vi "Horst-ECD.vi"() -> ()   [LabVIEW 2017]
uses:
  <vilib>/rvi/interface/nirviMethod/nirviMethod.xnode
  FPGA Bitfiles/HAGAR-VECD_FPGATarget_FPGA-ProgrammECD_J-wKM9Jb3G8.lvbitx
  E:/HAGAR-V_ECD/FPGA-Programm_ECD.vi
  <vilib>/rvi/errors/niLvFpgaMergeErrorWithErrorCode.vi
  <vilib>/FPGAPlugInAG/cRIO-9035/niLvFpga_ReadFifo_cRIO-9035.vi
  <vilib>/FPGAPlugInAG/cRIO-9035/niLvFpga_WriteFifo_cRIO-9035.vi
panel:
  in  "MWAntwortMod2":string[](array[string])=[":0622020121", ":0621020121", ":0626020121", ":0620020121", ":0624020121", ":0625020121", ":0623020121"]
  in  "MWabfragenMod2":string[](array[string])=[":06220401210120", ":06210401210120", ":06260401210120", ":06200401210120", ":06240401210120", ":06250401210120", ":06230401210120"]
  in  "FaktorMod2":dbl[](array[numeric])=[0.00625, 0.00625, 0.15625, 0.00015625, 0.00625, 0.00625, 0.00015625]
  in  "SPvorgebenMod2":string[](array[string])=[":0622010121", ":0621010121", ":0626010121", ":0620010121", ":0624010121", ":0625010121", ":0623010121"]
  in  "FPGA-VI-Referenz":refnum<k20>
  out "Array":errorcluster[](array[cluster])
  out "MW":dbl[](array[numeric])
  out "Fehler":bool[](array[boolean])
  in  "SP":dbl[](array[numeric]) format="%#_13g"
  in  "Stopp":bool
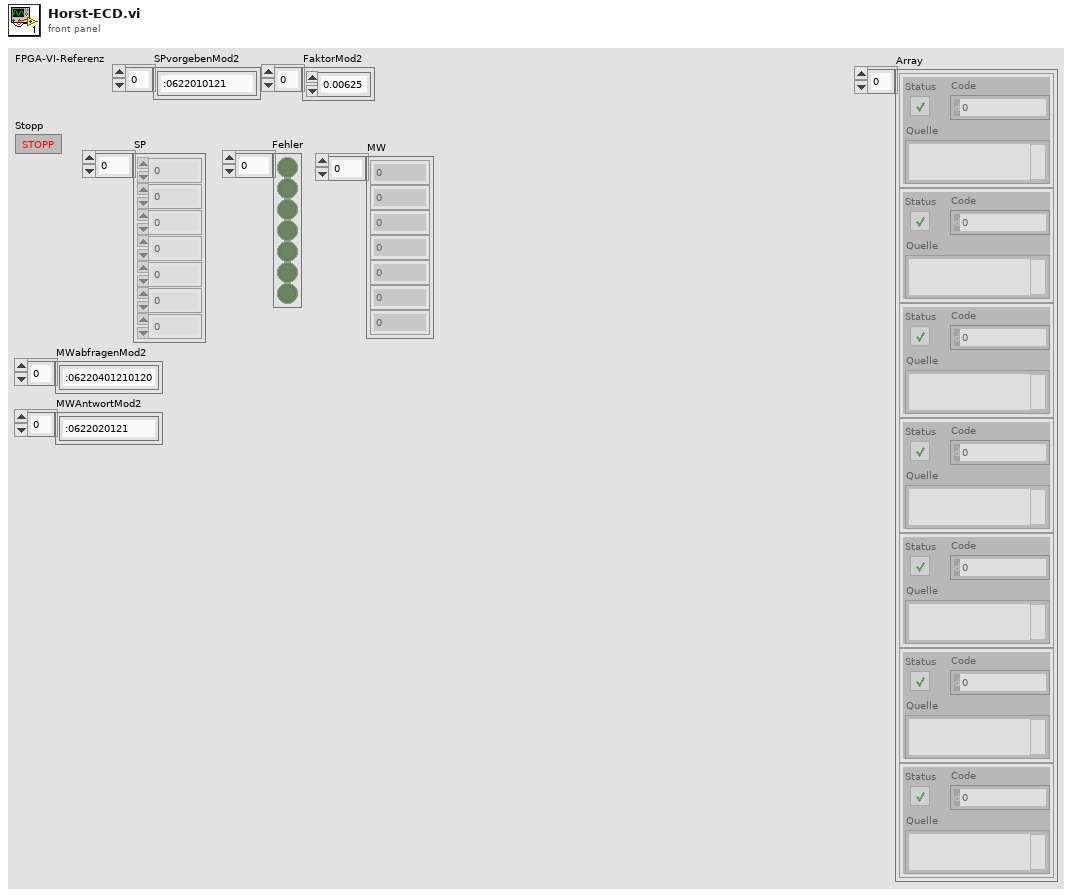
[diagram p1: front panel]
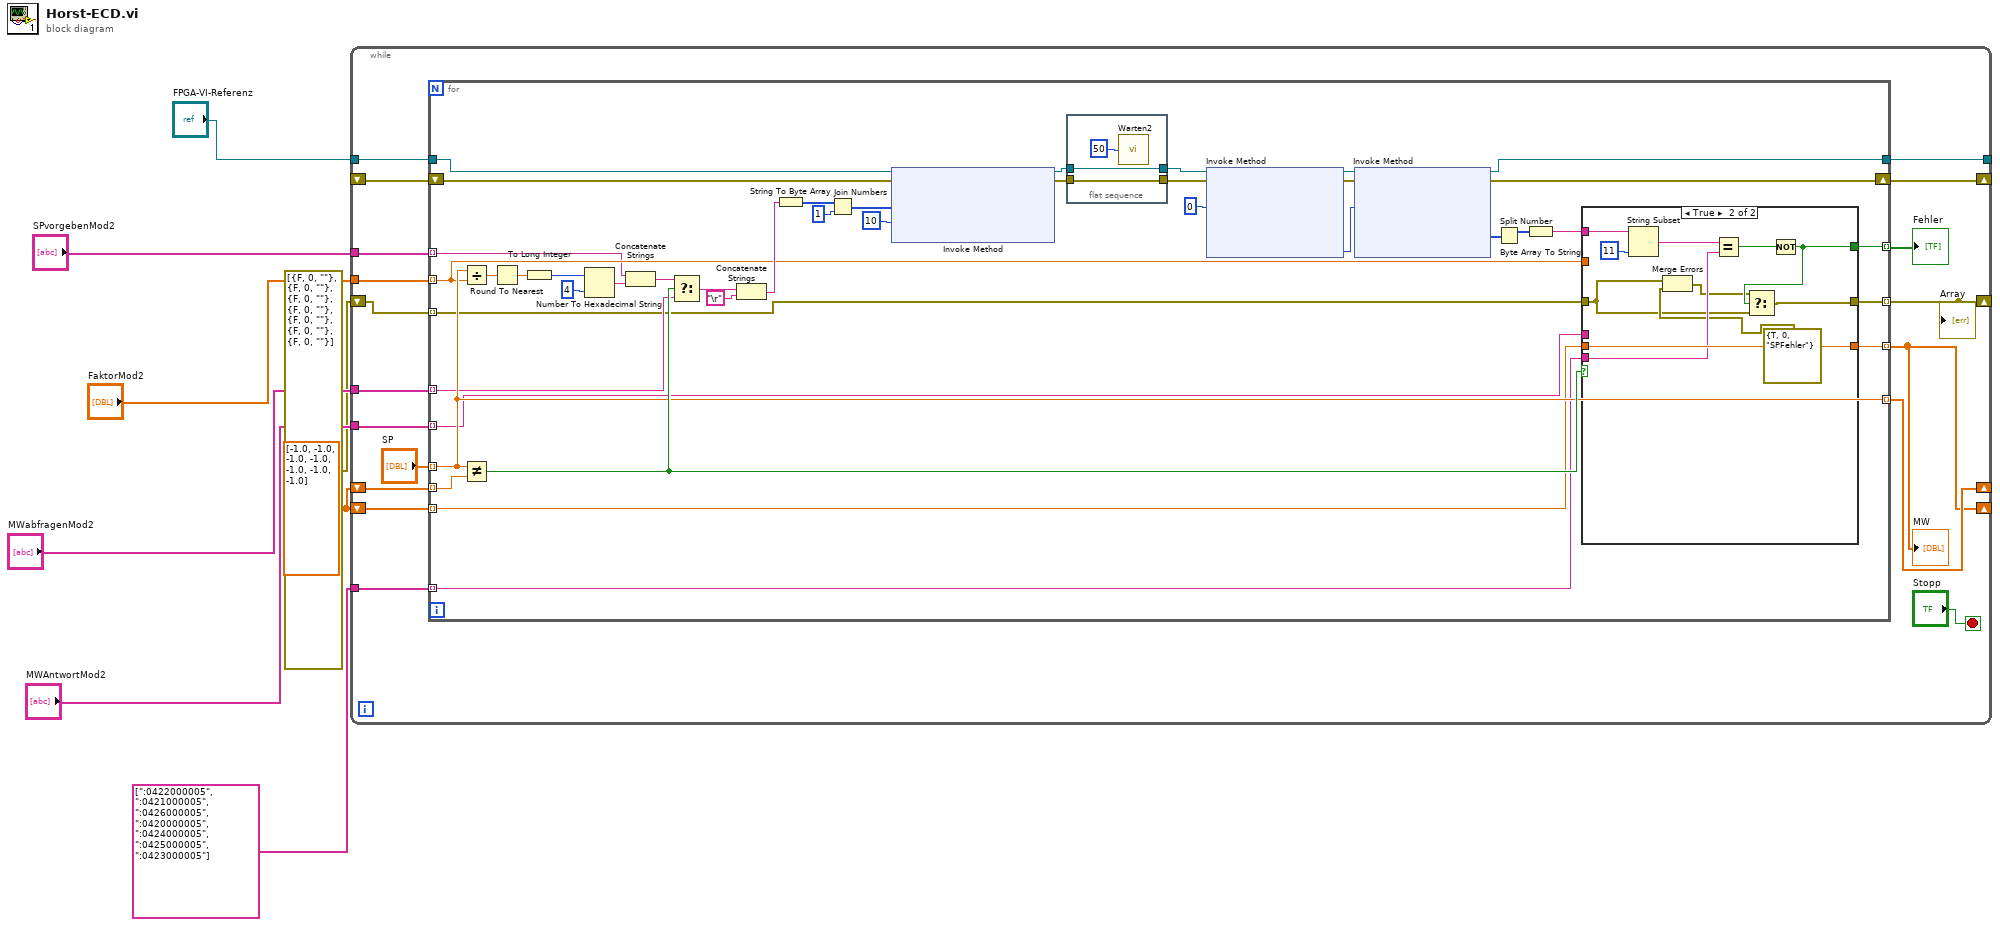
[diagram p0: block diagram]
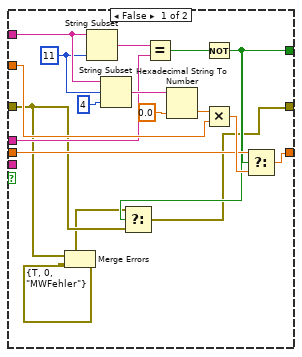
[diagram p2: hidden frame]
diagram:
  w8 = dbl[] [-1.0, -1.0, -1.0, -1.0, -1.0, -1.0, -1.0]
  n1 = while {
    shift-right: [w25] -> _
    shift-left: _ -> [w23]
    shift-right: [w20] -> _
    shift-left: w8 -> [w21]
    shift-right: [w17] -> _
    shift-left: w8 -> [w16]
    tunnel: "SPvorgebenMod2" -> [w15]
    tunnel: "MWabfragenMod2" -> [w14]
    tunnel: "FaktorMod2" -> [w13]
    tunnel: "MWAntwortMod2" -> [w12]
    tunnel: string[] [":0422000005", ":0421000005", ":0426000005", ":0420000005", ":0424000005", ":0425000005", ":0423000005"] ("y") -> [w11]
    shift-right: [w10] -> _
    shift-left: errorcluster[] [{"status"=FALSE, "code"=0, "source"=""}, {"status"=FALSE, "code"=0, "source"=""}, {"status"=FALSE, "code"=0, "source"=""}, {"status"=FALSE, "code"=0, "source"=""}, {"status"=FALSE, "code"=0, "source"=""}, {"status"=FALSE, "code"=0, "source"=""}, {"status"=FALSE, "code"=0, "source"=""}] -> [w9]
    tunnel: "FPGA-VI-Referenz" -> [w24]
    tunnel: [w26] -> _
    stop <- "Stopp" stop-if-true
    n2 = for {
      tunnel: w21 -> [w40] mode=indexing
      tunnel: [w36] -> w20 mode=indexing
      tunnel: [w37] -> w19 mode=indexing
      shift-right: [w60] -> w25
      shift-left: w23 -> [w52]
      tunnel: "SP" -> [w36] mode=indexing
      tunnel: w13 -> [w35] mode=indexing
      tunnel: [w34] -> w17 mode=indexing
      tunnel: w16 -> [w33] mode=indexing
      tunnel: w15 -> [w32] mode=indexing
      tunnel: w14 -> [w31] mode=indexing
      tunnel: w12 -> [w30] mode=indexing
      tunnel: w11 -> [w29] mode=indexing
      tunnel: [w28] -> w10 mode=indexing
      tunnel: w9 -> [w27] mode=indexing
      tunnel: w24 -> [w53]
      tunnel: [w63] -> w26
      n3 = Divide(x=w36, y=w35) -> (x/y=w47:dbl)
      n4 = Not Equal?(x=w36, y=w40) -> (x != y?=w38:bool)
      n5 = Round To Nearest(number=w47) -> (nearest integer value=w46:dbl)
      n6 = To Long Integer(number=w46) -> (32bit integer=w45:i32)
      n7 = Number To Hexadecimal String(1:i16 4 ("Breite (-)"), 2:w45) -> (0:w43:string)
      n8 = Concatenate Strings(w32, w43) -> (w42:string)
      n9 = Select(t=w42, s=w38, f=w31) -> (s? t:f=w41:string)
      n10 = Concatenate Strings(w41, "\r") -> (w59:string)
      n11 = String To Byte Array(string=w59) -> (unsigned byte array=w57:u8[])
      n12 = Join Numbers(hi=w57, lo=u8 1) -> ((hi.lo)=w58:u16[])
      n13 = xnode "Invoke Method"("FPGA-VI-Referenz (Eingang)"=w53, "Fehler (Eingang)"=w52, "Daten"=w58, "Timeout (ms)"=10) -> ("FPGA-VI-Referenz (Ausgang)"=w51:refnum<k20>, "Fehler (Ausgang)"=w49:errorcluster)  [unwired: 1 out]
      n14 = flat-sequence {
        tunnel: w51 -> [w99]
        tunnel: [w99] -> w50
        tunnel: w49 -> [w98]
        tunnel: [w98] -> w48
        frame #0 {
          n15 = call "Warten2"("Count(mSec)"=u32 50) -> ()  [unwired: 1 out]
        }
      }
      n16 = xnode "Invoke Method"("FPGA-VI-Referenz (Eingang)"=w50, "Fehler (Eingang)"=w48, "Anzahl der Elemente"=u32 0) -> ("FPGA-VI-Referenz (Ausgang)"=w62:refnum<k20>, "Fehler (Ausgang)"=w61:errorcluster, "Verbleibende Elemente"=w66:u32)  [unwired: 1 in, 1 out]
      n17 = xnode "Invoke Method"("FPGA-VI-Referenz (Eingang)"=w62, "Fehler (Eingang)"=w61, "Anzahl der Elemente"=w66) -> ("FPGA-VI-Referenz (Ausgang)"=w63:refnum<k20>, "Fehler (Ausgang)"=w60:errorcluster, "Daten"=w65:u16[])  [unwired: 1 in, 1 out]
      n18 = Split Number(x=w65) -> (hi(x)=w64:u8[])  [unwired: 1 out]
      n19 = Byte Array To String(unsigned byte array=w64) -> (string=w39:string)
      n20 = case shown="True" w38 {
        tunnel: w39 -> [w83 w96]
        tunnel: [w72 w90] -> w37
        tunnel: w35 -> [w77 _]
        tunnel: [w74 w92] -> w34
        tunnel: w33 -> [w75 w92]
        tunnel: w30 -> [w73 _]
        tunnel: w29 -> [_ w91]
        tunnel: [w71 w89] -> w28
        tunnel: w27 -> [w70 w86]
        frame False {
          w82 = 11 ("Länge (Rest)")
          n21 = Merge Errors(w70, errorcluster {"status"=TRUE, "code"=0, "source"="MWFehler"} ("Fehlerkonstante")) -> (w69:errorcluster)
          n22 = String Subset(string=w83, length (rest)=w82) -> (substring=w85:string)  [unwired: 1 in]
          n23 = String Subset(string=w83, offset (0)=w82, length (rest)=4 ("Länge (Rest)")) -> (substring=w80:string)
          n24 = Equal?(x=w85, y=w73) -> (x = y?=w84:bool)
          n25 = Hexadecimal String To Number(string=w80, default (0uL)=0.0 ("Standard (0 U32)")) -> (number=w78:dbl)  [unwired: 1 in, 1 out]
          n26 = Not(x=w84) -> (.not. x?=w72:bool)
          n27 = Select(t=w69, s=w72, f=w70) -> (s? t:f=w71:errorcluster)
          n28 = Multiply(x=w78, y=w77) -> (x*y=w76:dbl)
          n29 = Select(t=w75, s=w72, f=w76) -> (s? t:f=w74:dbl)
        }
        frame True {
          n30 = String Subset(string=w96, length (rest)=11 ("Länge (Rest)")) -> (substring=w95:string)  [unwired: 1 in]
          n31 = Merge Errors(w86, errorcluster {"status"=TRUE, "code"=0, "source"="SPFehler"} ("Fehler (Eingang)")) -> (w87:errorcluster)
          n32 = Equal?(x=w95, y=w91) -> (x = y?=w93:bool)
          n33 = Not(x=w93) -> (.not. x?=w90:bool)
          n34 = Select(t=w87, s=w90, f=w86) -> (s? t:f=w89:errorcluster)
        }
      }
    }
    "Fehler" <- w19
    "MW" <- w17
    "Array" <- w10
  }
